vi "FileReadSearch.vi"() -> ()   [LabVIEW 2021]
panel:
  out "Count":i16
  in  "Alphabet to count":string
  out "String Characters":i32
  out "text":string
  in  "Path":path
  out "error out":errorcluster
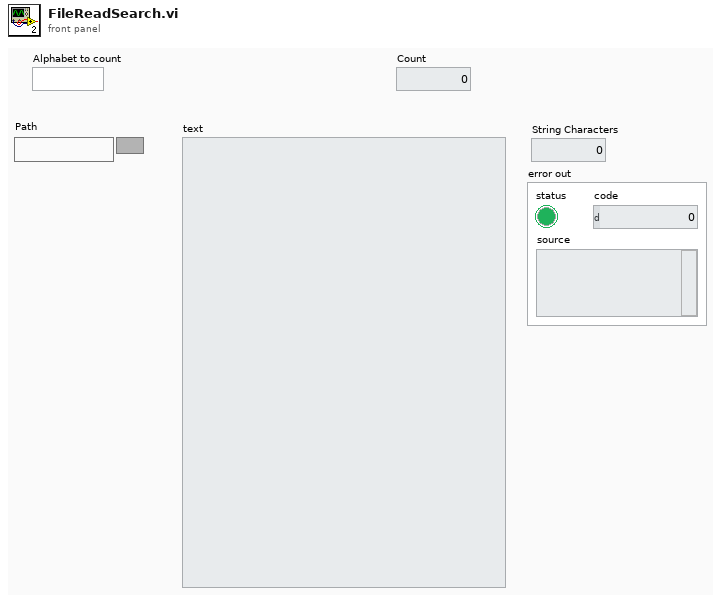
[diagram p1: front panel]
types:
  T1 = enum16{"open", "replace", "create", "open or create", "replace or create", "replace or create with confirmation"}
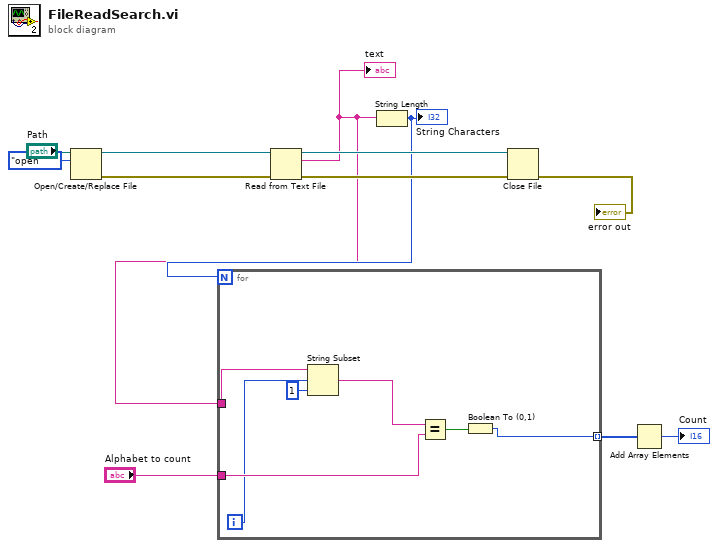
[diagram p0: block diagram]
diagram:
  n1 = Open/Create/Replace File(file path (use dialog)="Path", operation (0:open)=T1."open") -> (refnum out=w12:refnum<file>, error out=w10:errorcluster)  [unwired: 4 in, 1 out]
  n2 = Read from Text File(file (use dialog)=w12, error in=w10) -> (refnum out=w11:refnum<file>, text=w4:string, error out=w9:errorcluster)  [unwired: 2 in, 1 out]
  "text" <- w4
  n3 = String Length(string=w4) -> (length=w5:i32)
  "String Characters" <- w5
  n4 = for {
    N: w5 -> [_]
    tunnel: w4 -> [w19]
    tunnel: "Alphabet to count" -> [w16]
    tunnel: [w14] -> w2 mode=indexing
    i -> [w13]
    n5 = String Subset(string=w19, offset (0)=w13, length (rest)=1 ("length (rest)")) -> (substring=w17:string)
    n6 = Equal?(x=w17, y=w16) -> (x = y?=w15:bool)
    n7 = Boolean To (0,1)(Boolean=w15) -> (0, 1=w14:i16)
  }
  n8 = Close File(refnum=w11, error in=w9) -> (error out=→"error out":errorcluster)  [unwired: 1 out]
  n9 = Add Array Elements(numeric array=w2) -> (sum=→"Count":i16)
